vi "MCL Iss Bind Clock To Axis.vi"(7 "handle":i32, 9 "axis":i32, 10 "mode":i32, 11 "clock":i32) -> (3 "function return":i32)   [LabVIEW 2017, in "Madlib.lvlib"]
doc: "MADLIB_API int MCL_IssBindClockToAxis(int clock, int mode, int axis, int handle);"
uses:
  Madlib.lvlib
  Madlib.dll
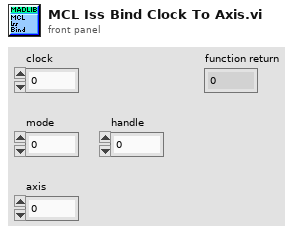
[diagram p1: front panel]
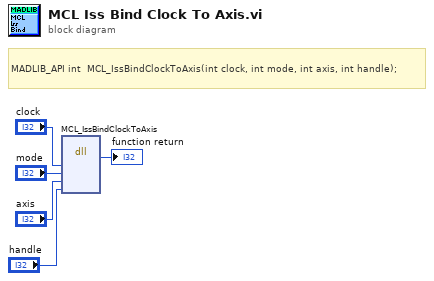
[diagram p0: block diagram]
diagram:
  # "MADLIB_API\tint\t\tMCL_IssBindClockToAxis(int clock, int mode, int axis, int handle);"
  n1 = dll-call lib="C:/Users/francesco/dev/pump-probe/Piezo/lvlib/Madlib.*" fn="MCL_IssBindClockToAxis"("clock"="clock", "mode"="mode", "axis"="axis", "handle"="handle") -> (→"function return":i32)  [unwired: 7 in, 2 out]
